vi "Run Test Application.vi"(8 "error in (no error)":errorcluster, 10 "Tests":refnum<class "Test Class.lvclass">[](array[class]), 11 "Application in":refnum<class "Application.lvclass">) -> (0 "error out":errorcluster, 3 "Application out":refnum<class "Application.lvclass">)   [LabVIEW 2017, in "Application.lvlib" / "Application.lvclass"]
uses:
  Application.lvclass
  Tests/Test Class/Test Class.lvclass
  <vilib>/TSS/ACRObat Test Framework/Core Launcher/Core Manager Methods -- Enum.ctl
  <vilib>/TSS/ACRObat Test Framework/Core Launcher/Core Launcher.lvlib
  <vilib>/TSS/ACRObat Test Framework/Classes/Data/Data Repo/Class/Data Repo.lvclass
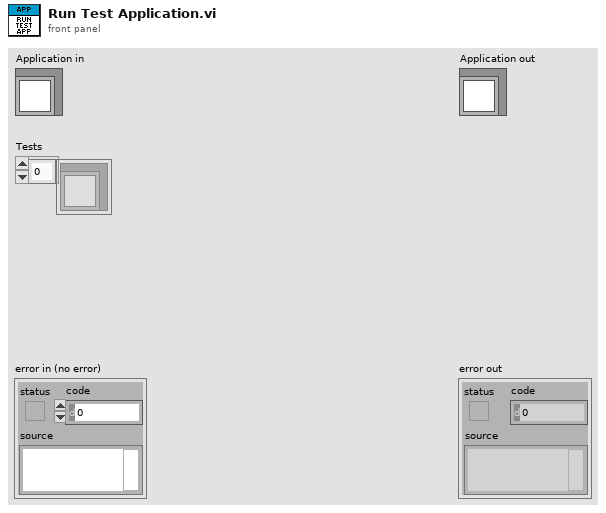
[diagram p1: front panel]
types:
  T1 = typedef "Core Launcher.lvlib/Core Manager Methods -- Enum.ctl" = enum16{"Spawn Objects", "Get Objects", "Destroy Objects"}
  T2 = cluster{"Serial Number Reference":refnum<vi>, "Status Message Reference":refnum<vi>, "Position":u32}[]
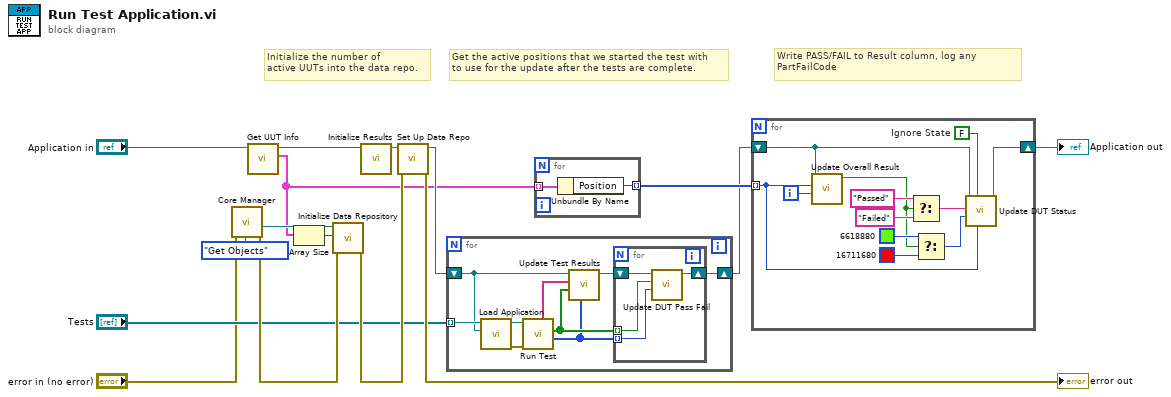
[diagram p0: block diagram]
diagram:
  # "Write PASS/FAIL to Result column, log any PartFailCode"
  # "Get the active positions that we started the test with \nto use for the update after the tests are complete."
  # "Initialize the number of\nactive UUTs into the data repo."
  n1 = call <vilib>:"Core Manager.vi"("Method"=Core_Manager_Methods_--_Enum."Get Objects", "error in (no error)"="error in (no error)") -> ("error out"=w12:errorcluster, "Data Repo"=w15:refnum<class "Data Repo.lvclass">)  [unwired: 5 in, 3 out]
  n2 = call-dynamic "Get UUT Info.vi"("Application in"="Application in") -> ("All UUTs"=w1:T2, "Application out"=w3:refnum<class "Application.lvclass">)  [unwired: 8 in, 1 out]
  n3 = Array Size(array=w1) -> (size(s)=w9:i32)
  n4 = call <vilib>:"Initialize Data Repository.vi"("error in (no error)"=w12, "Number of DUTs"=w9, "Acrobat Template in"=w15) -> ("error out"=w13:errorcluster)  [unwired: 7 in, 1 out]
  n5 = call "Initialize Results.vi"("Application in"=w3) -> ("Application out"=w6:refnum<class "Application.lvclass">)  [unwired: 9 in, 1 out]
  n6 = call "Set Up Data Repo.vi"("error in (no error)"=w13, "Application in"=w6) -> ("error out"=→"error out":errorcluster, "Application out"=w14:refnum<class "Application.lvclass">)  [unwired: 8 in]
  n7 = for {
    tunnel: "Tests" -> [w25] mode=indexing
    shift-right: [w19] -> w5
    shift-left: w14 -> [w22]
    n8 = call "Load Application.vi"("Application.lvlib:Application.lvclass"=w22, "Test Class in"=w25) -> ("error out"=w23:errorcluster, "Test Class out"=w24:refnum<class "Test Class.lvclass">)  [unwired: 8 in]
    n9 = call-dynamic "Run Test.vi"("error in (no error)"=w23, "Test Class in"=w24) -> ("Positions"=w17:i32[], "Tests Passed"=w18:bool[], "Fail Codes"=w21:string[])  [unwired: 5 in, 2 out]
    n10 = call "Update Test Results.vi"("Positions"=w17, "Tests Passed"=w18, "Fail Codes"=w21, "Application in"=w22) -> ("Application in"=w20:refnum<class "Application.lvclass">)  [unwired: 6 in, 1 out]
    n11 = for {
      shift-right: [w28] -> w19
      shift-left: w20 -> [w29]
      tunnel: w18 -> [w27] mode=indexing
      tunnel: w17 -> [w26] mode=indexing
      n12 = call "Update DUT Pass Fail.vi"("Position"=w26, "Test Passed"=w27, "Application in"=w29) -> ("Application out"=w28:refnum<class "Application.lvclass">)  [unwired: 7 in, 1 out]
    }
  }
  n13 = for {
    tunnel: w1 -> [w31] mode=indexing
    tunnel: [w30] -> w8 mode=indexing
    n14 = Unbundle By Name(w31) -> ("Position"=w30:u32)
  }
  n15 = for {
    shift-right: [w34] -> w7
    shift-left: w5 -> [w37]
    tunnel: w8 -> [w33] mode=indexing
    i -> [w36]
    w38 = FALSE  # Ignore State
    n16 = call "Update Overall Result.vi"("Data Row"=w36, "Position"=w33, "Application in"=w37) -> ("Pass"=w35:bool)  [unwired: 8 in]
    n17 = Select(t="Passed", s=w35, f="Failed") -> (s? t:f=w32:string)
    n18 = Select(t=u32 6618880, s=w35, f=u32 16711680) -> (s? t:f=w39:u32)
    n19 = call "Update DUT Status.vi"("Position"=w33, "Ignore State (true)"=w38, "BG Color"=w39, "Message ('')"=w32, "Application in"=w37) -> ("Application out"=w34:refnum<class "Application.lvclass">)  [unwired: 5 in, 1 out]
  }
  "Application out" <- w7
